vi "TagMetadataToImage.vi"(8 "error in (no error)":errorcluster, 10 "Image In":T1, 11 "DemoStepMotor in":refnum<class "DemoStepMotor.lvclass">) -> (0 "error out":errorcluster, 2 "Image Out":T1, 3 "DemoStepMotor out":refnum<class "DemoStepMotor.lvclass">)   [LabVIEW 2020, in "DemoStepMotor.lvlib" / "DemoStepMotor.lvclass"]
uses:
  DemoStepMotor.lvclass
  <vilib>/vision/Image Controls.llb/IMAQ Image.ctl
  DemoStepMotor.lvclass/DemoStepMotor.ctl
  Hardware Abstraction Layer/Component/Stage/Stage/Stage.lvclass
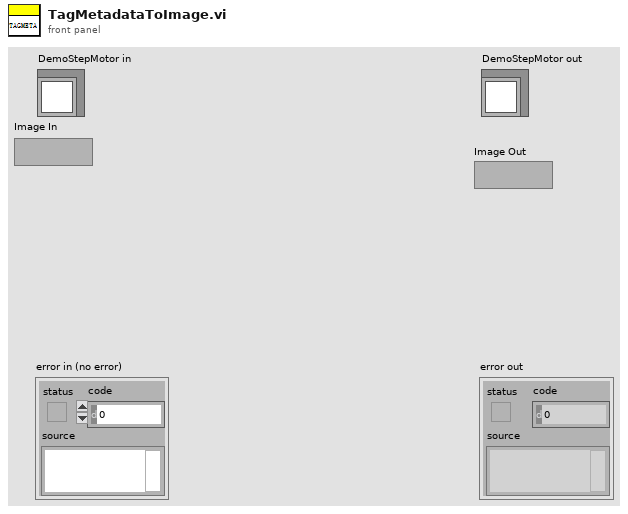
[diagram p1: front panel]
types:
  T1 = typedef "IMAQ Image.ctl" = refnum<image>
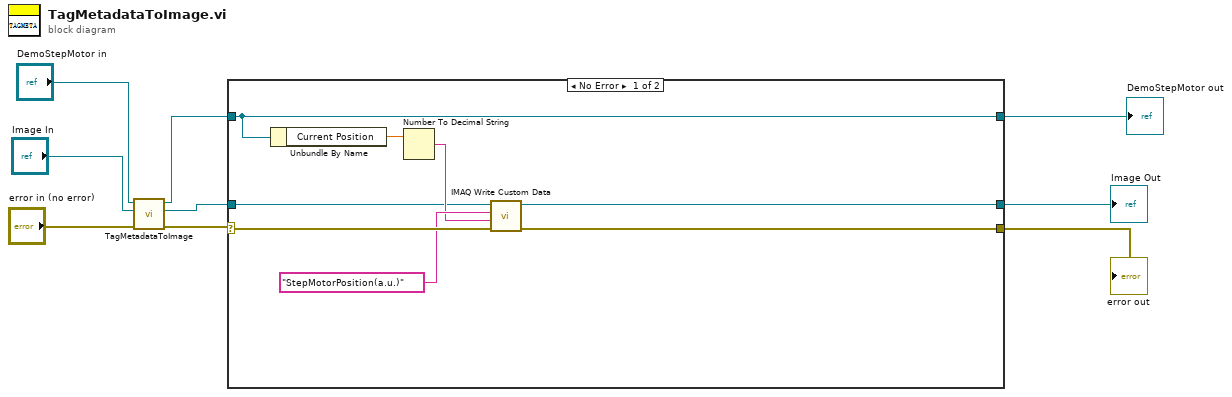
[diagram p0: block diagram]
diagram:
  n1 = call-parent "TagMetadataToImage.vi"("error in (no error)"="error in (no error)", "Image In"="Image In", "Device in"="DemoStepMotor in") -> ("error out"=w6:errorcluster, "Image Out"=w4:T1, "Device out"=w2:refnum<class "DemoStepMotor.lvclass">)  [unwired: 6 in]
  n2 = case shown="No Error" w6 {
    selector: w6 -> [w15 w20]
    tunnel: [w14 w20] -> w5
    tunnel: w4 -> [w11 w19]
    tunnel: [w10 w19] -> w3
    tunnel: [w17 w18] -> w1
    tunnel: w2 -> [w17 w18]
    frame No Error {
      n3 = Unbundle By Name(w17) -> ("Current Position"=w16:dbl)
      n4 = Number To Decimal String(number=w16) -> (decimal integer string=w12:string)  [unwired: 1 in]
      n5 = call "IMAQ Write Custom Data"("error in (no error)"=w15, "Custom Data In"=w12, "Key"="StepMotorPosition(a.u.)", "Image"=w11) -> ("error out"=w14:errorcluster, "Image Out"=w10:T1)  [unwired: 6 in]
    }
    frame Error {
    }
  }
  "error out" <- w5
  "DemoStepMotor out" <- w1
  "Image Out" <- w3
